vi "niDAQmx Read.vi"   [LabVIEW 2021, in "Session Management niDAQmx.lvlib" / "Session Factory.lvclass"]
doc: "Reads samples from the task or virtual channels you specify. The instances of this polymorphic VI specify what format of samples to return, whether to read a single sample or multiple samples at once, and whether to read from one or multiple channels."
uses:
  Session Factory.lvclass
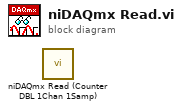
[diagram p0: block diagram]
diagram:
  n1 = call "niDAQmx Read (Counter DBL 1Chan 1Samp).vi"() -> ()  [unwired: 13 in, 3 out]
